vi "milliGAT Letter the Enum.vi"(10 "Pump Letter":string, 11 "Enum in":refnum<vi>) -> (3 "Numeric":i32)   [LabVIEW 2018, in "VICI M6 M50 Party Mode.lvlib"]
uses:
  VICI M6 M50 Party Mode.lvlib
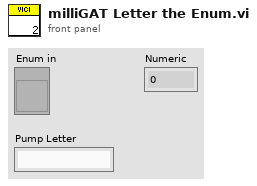
[diagram p1: front panel]
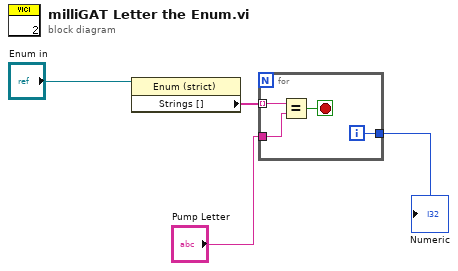
[diagram p0: block diagram]
diagram:
  n1 = property on="Property Node" class="Enum (strict)"(reference="Enum in") -> ("Strings []"=w3:string[])  [unwired: 1 in, 2 out]
  n2 = for {
    tunnel: w3 -> [w8] mode=indexing
    tunnel: "Pump Letter" -> [w7]
    tunnel: [w5] -> w1
    i -> [w5]
    stop <- w6 stop-if-true
    n3 = Equal?(x=w8, y=w7) -> (x = y?=w6:bool)
  }
  "Numeric" <- w1
